vi "Load Stimulus Parameters (SubVI).vi"(11 "Stimulus File Name":path=path "C:/MWT/Config.ini") -> (0 "STIM MODE":string, 3 "STIM Param":dbl[](array[numeric]))   [LabVIEW 2020]
uses:
  Controls (HOST)/Stimulus Param.ctl
  <vilib>/Utility/config.llb/Read Key (Double).vi
  <vilib>/Utility/config.llb/Read Key (String).vi
  <vilib>/Utility/config.llb/NI_LVConfig.lvlib
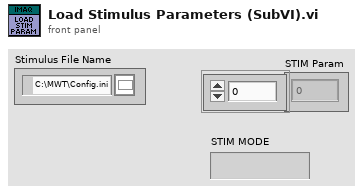
[diagram p1: front panel]
types:
  T1 = typedef "Stimulus Param.ctl" = enum16{"STIM 1", "STIM 2", "STIM 3", "STIM 4", "STIM 5", "STIM 6", "STIM 7", "STIM 8", "STIM 9", "STIM 10"}
  T2 = typedef "NI_LVConfig.lvlib/Config Data RefNum.ctl" = refnum<k1>
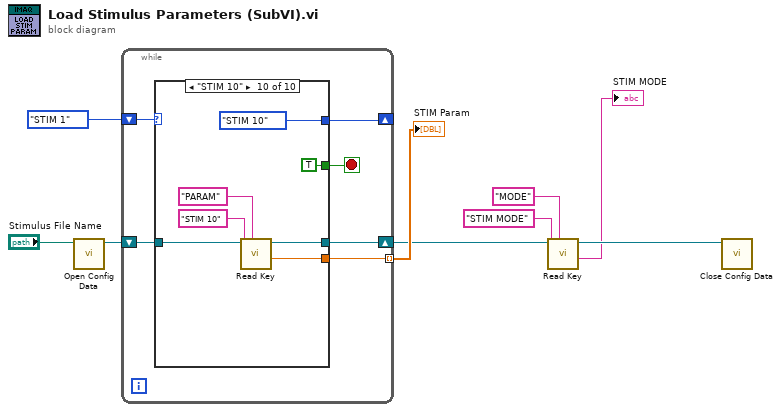
[diagram p0: block diagram]
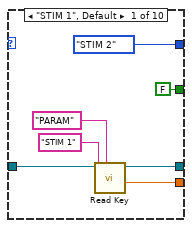
[diagram p2: hidden frame]
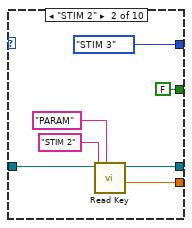
[diagram p3: hidden frame]
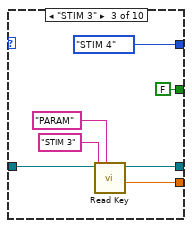
[diagram p4: hidden frame]
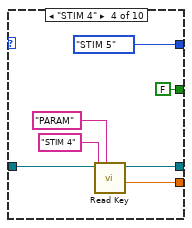
[diagram p5: hidden frame]
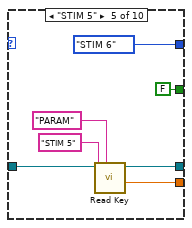
[diagram p6: hidden frame]
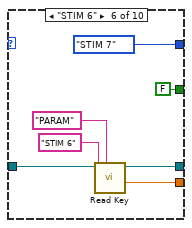
[diagram p7: hidden frame]
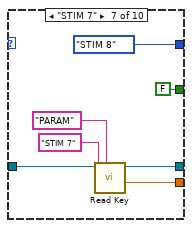
[diagram p8: hidden frame]
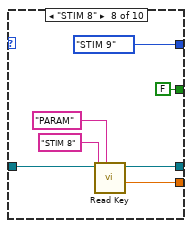
[diagram p9: hidden frame]
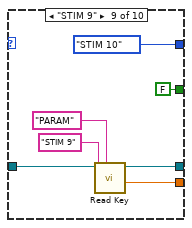
[diagram p10: hidden frame]
diagram:
  n1 = call <vilib>:"Open Config Data.vi"("configuration file path"="Stimulus File Name") -> ("refnum"=w9:T2)  [unwired: 8 in, 2 out]
  n2 = while {
    shift-right: [w14] -> w3
    shift-left: w9 -> [w15]
    shift-right: [w11] -> _
    shift-left: Stimulus_Param."STIM 1" -> [w13]
    tunnel: [w10] -> w6 mode=indexing
    stop <- w12 stop-if-true
    n3 = case shown="\"STIM 10\"" w13 {
      tunnel: w15 -> [w22 w29 w36 w43 w50 w57 w64 w71 w78 w85]
      tunnel: [w21 w28 w35 w42 w49 w56 w63 w70 w77 w84] -> w14
      tunnel: [FALSE FALSE FALSE FALSE FALSE FALSE FALSE FALSE FALSE TRUE] -> w12
      tunnel: [Stimulus_Param."STIM 2" Stimulus_Param."STIM 3" Stimulus_Param."STIM 4" Stimulus_Param."STIM 5" Stimulus_Param."STIM 6" Stimulus_Param."STIM 7" Stimulus_Param."STIM 8" Stimulus_Param."STIM 9" Stimulus_Param."STIM 10" Stimulus_Param."STIM 10"] -> w11
      tunnel: [w16 w23 w30 w37 w44 w51 w58 w65 w72 w79] -> w10
      frame "STIM 1", Default {
        n4 = call-poly <vilib>:"Read Key.vi"("section"="PARAM", "key"="STIM 1" ("section"), "refnum"=w22) -> ("value"=w16:dbl, "refnum out"=w21:T2)  [unwired: 5 in, 2 out]
      }
      frame "STIM 2" {
        n5 = call-poly <vilib>:"Read Key.vi"("section"="PARAM", "key"="STIM 2" ("section"), "refnum"=w29) -> ("value"=w23:dbl, "refnum out"=w28:T2)  [unwired: 5 in, 2 out]
      }
      frame "STIM 3" {
        n6 = call-poly <vilib>:"Read Key.vi"("section"="PARAM", "key"="STIM 3" ("section"), "refnum"=w36) -> ("value"=w30:dbl, "refnum out"=w35:T2)  [unwired: 5 in, 2 out]
      }
      frame "STIM 4" {
        n7 = call-poly <vilib>:"Read Key.vi"("section"="PARAM", "key"="STIM 4" ("section"), "refnum"=w43) -> ("value"=w37:dbl, "refnum out"=w42:T2)  [unwired: 5 in, 2 out]
      }
      frame "STIM 5" {
        n8 = call-poly <vilib>:"Read Key.vi"("section"="PARAM", "key"="STIM 5" ("section"), "refnum"=w50) -> ("value"=w44:dbl, "refnum out"=w49:T2)  [unwired: 5 in, 2 out]
      }
      frame "STIM 6" {
        n9 = call-poly <vilib>:"Read Key.vi"("section"="PARAM", "key"="STIM 6" ("section"), "refnum"=w57) -> ("value"=w51:dbl, "refnum out"=w56:T2)  [unwired: 5 in, 2 out]
      }
      frame "STIM 7" {
        n10 = call-poly <vilib>:"Read Key.vi"("section"="PARAM", "key"="STIM 7" ("section"), "refnum"=w64) -> ("value"=w58:dbl, "refnum out"=w63:T2)  [unwired: 5 in, 2 out]
      }
      frame "STIM 8" {
        n11 = call-poly <vilib>:"Read Key.vi"("section"="PARAM", "key"="STIM 8" ("section"), "refnum"=w71) -> ("value"=w65:dbl, "refnum out"=w70:T2)  [unwired: 5 in, 2 out]
      }
      frame "STIM 9" {
        n12 = call-poly <vilib>:"Read Key.vi"("section"="PARAM", "key"="STIM 9" ("section"), "refnum"=w78) -> ("value"=w72:dbl, "refnum out"=w77:T2)  [unwired: 5 in, 2 out]
      }
      frame "STIM 10" {
        n13 = call-poly <vilib>:"Read Key.vi"("section"="PARAM", "key"="STIM 10" ("section"), "refnum"=w85) -> ("value"=w79:dbl, "refnum out"=w84:T2)  [unwired: 5 in, 2 out]
      }
    }
  }
  "STIM Param" <- w6
  n14 = call-poly <vilib>:"Read Key.vi"("section"="MODE", "key"="STIM MODE" ("section"), "refnum"=w3) -> ("value"=→"STIM MODE":string, "refnum out"=w2:T2)  [unwired: 5 in, 2 out]
  n15 = call <vilib>:"Close Config Data.vi"("refnum"=w2) -> ()  [unwired: 9 in, 2 out]
